vi "Auton Scripting.vi"   [LabVIEW 2014]
uses:
  <vilib>/Rock Robotics/WPI/DriverStation/WPI_DriverStationRobotMode2.ctl
  Begin/Global Variables.vi
types:
  T1 = typedef "WPI_DriverStationRobotMode2.ctl" = enum16{"Autonomous Disabled", "Autonomous Enabled", "Teleop Disabled", "Teleop Enabled", "Disconnected", "Finish", "Test Disabled", "Test Enabled", "Emergency Stopped"}
  T2 = cluster{"primitive":i32, "argument 1":dbl, "argument 2":dbl, "argument 3":dbl, "argument 4":dbl, "argument 5":dbl}
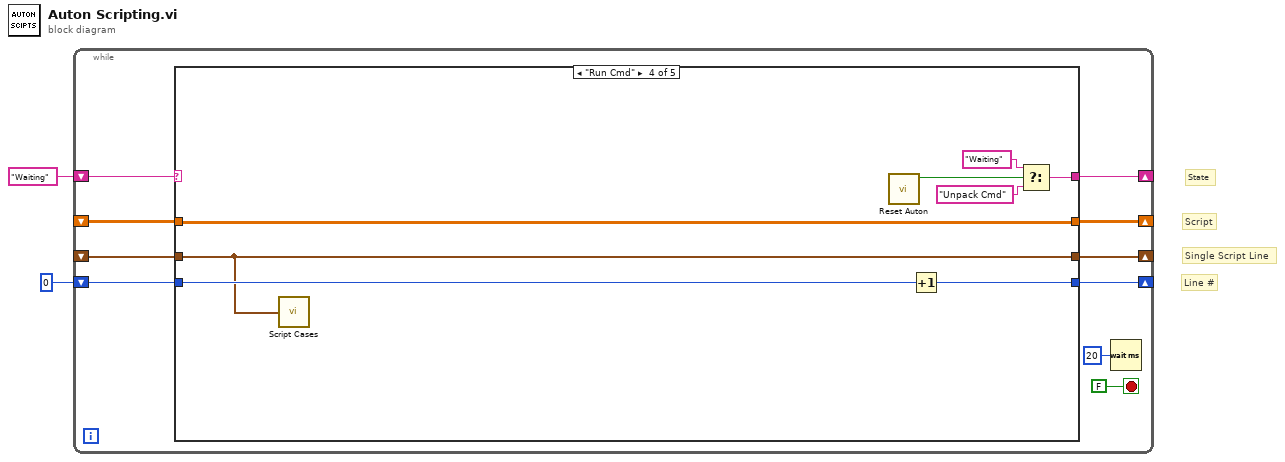
[diagram p0: block diagram]
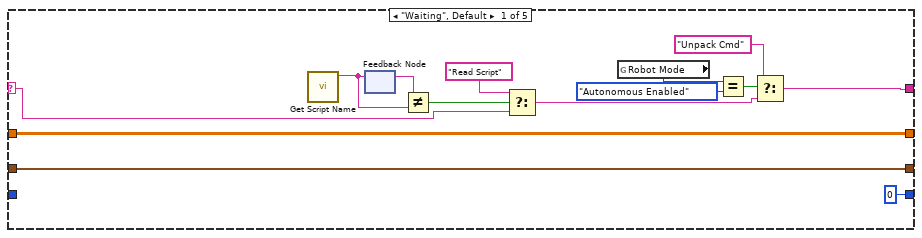
[diagram p2: hidden frame]
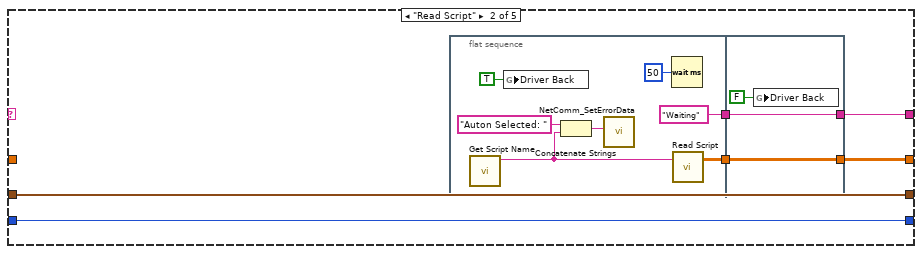
[diagram p3: hidden frame]
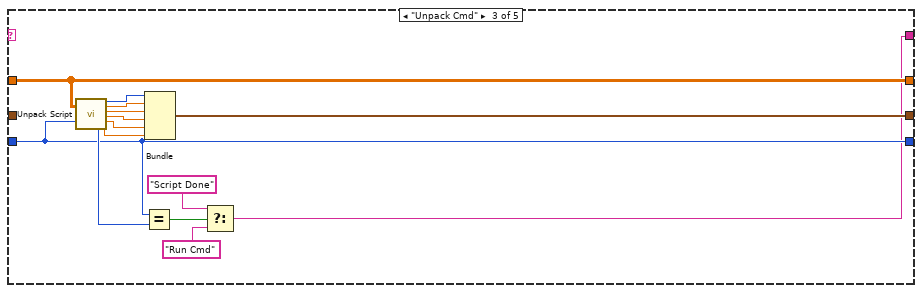
[diagram p4: hidden frame]
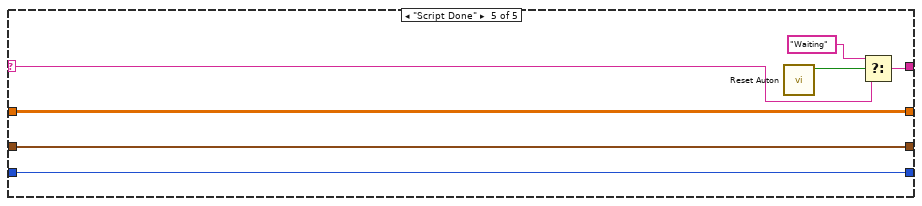
[diagram p5: hidden frame]
diagram:
  # "Line #"
  # "Single Script Line"
  # "Script"
  # "State"
  n1 = while {
    shift-right: [w10] -> _
    shift-left: "Waiting" ("Name") -> [w11]
    shift-right: [w9] -> _
    shift-left: _ -> [w8]
    shift-right: [w7] -> _
    shift-left: _ -> [w4]
    shift-right: [w5] -> _
    shift-left: u32 0 ("milliseconds to wait") -> [w6]
    stop <- FALSE stop-if-true
    n2 = case shown="\"Run Cmd\"" w11 {
      selector: w11 -> [w14 _ _ _ w68]
      tunnel: [w16 w31 w43 w62 w71] -> w10
      tunnel: [w22 w32 w49 w61 w67] -> w9
      tunnel: w8 -> [w22 _ w49 w61 w67]
      tunnel: [w15 w29 w50 w57 w66] -> w7
      tunnel: w6 -> [_ w30 w47 w59 w65]
      tunnel: [u32 0 ("milliseconds to wait") w30 w47 w58 w65] -> w5
      tunnel: w4 -> [w15 w29 _ w57 w66]
      frame "Waiting", Default {
        n3 = call "Get Script Name.vi"() -> ("Script Name"=w26:string)  [unwired: 11 in]
        n4 = feedback-in #1(w26) -> ()
        n5 = feedback #1() -> (w25:string)  [unwired: 1 in]
        n6 = Not Equal?(x=w25, y=w26) -> (x != y?=w24:bool)
        n7 = Select(t="Read Script" ("Name"), s=w24, f=w14) -> (s? t:f=w21:string)
        n8 = global read "Global Variables.vi" "Robot Mode"() -> (w19:T1)
        n9 = Equal?(x=w19, y=WPI_DriverStationRobotMode2."Autonomous Enabled") -> (x = y?=w20:bool)
        n10 = Select(t="Unpack Cmd" ("Name"), s=w20, f=w21) -> (s? t:f=w16:string)
      }
      frame "Read Script" {
        n11 = flat-sequence {
          tunnel: [w39] -> w28
          tunnel: ["Waiting" ("Name")] -> w27
          tunnel: [w41] -> w31
          tunnel: [w42] -> w32
          tunnel: w28 -> [w42]
          tunnel: w27 -> [w41]
          frame #0 {
            n12 = call "Get Script Name.vi"() -> ("Script Name"=w36:string)  [unwired: 11 in]
            n13 = global write "Global Variables.vi" "Driver Back"(TRUE ("Driver Back")) -> ()
            n14 = Concatenate Strings("Auton Selected: " ("string"), w36) -> (w37:string)
            n15 = call <vilib>:"NetComm_SetErrorData.vi"("Error Data"=w37) -> ()  [unwired: 3 in, 8 out]
            n16 = Wait (ms)(milliseconds to wait=u32 50) -> ()  [unwired: 1 out]
            n17 = call "Read Script.vi"("script name"=w36) -> ("output array"=w39:dbl[][])  [unwired: 1 in, 1 out]
          }
          frame #1 {
            n18 = global write "Global Variables.vi" "Driver Back"(FALSE ("Driver Back")) -> ()
          }
        }
      }
      frame "Unpack Cmd" {
        n19 = call "Unpack Script.vi"("script"=w49, "index"=w47) -> ("# of primitives"=w48:i32, "primitive"=w56:i32, "argument 1"=w55:dbl, "argument 2"=w54:dbl, "argument 3"=w53:dbl, "argument 4"=w52:dbl, "argument 5"=w51:dbl)  [unwired: 11 in]
        n20 = Equal?(x=w47, y=w48) -> (x = y?=w46:bool)
        n21 = Bundle("primitive"=w56, "argument 1"=w55, "argument 2"=w54, "argument 3"=w53, "argument 4"=w52, "argument 5"=w51) -> (w50:T2)  [unwired: 1 in]
        n22 = Select(t="Script Done" ("Name"), s=w46, f="Run Cmd" ("Name")) -> (s? t:f=w43:string)
      }
      frame "Run Cmd" {
        n23 = call "Script Cases.vi"("Primitives & Arguments"=w57) -> ()
        n24 = call "Reset Auton.vi"() -> ("Reset Auton"=w60:bool)  [unwired: 11 in]
        n25 = Increment(x=w59) -> (x+1=w58:u32)
        n26 = Select(t="Waiting" ("Name"), s=w60, f="Unpack Cmd" ("Name")) -> (s? t:f=w62:string)
      }
      frame "Script Done" {
        n27 = call "Reset Auton.vi"() -> ("Reset Auton"=w70:bool)  [unwired: 11 in]
        n28 = Select(t="Waiting" ("Name"), s=w70, f=w68) -> (s? t:f=w71:string)
      }
    }
    n29 = Wait (ms)(milliseconds to wait=u32 20) -> ()  [unwired: 1 out]
  }
